vi "OAT DC Gap Estimator (1 Channel).vi"(0 "even-angle signal":cluster{"r0":dbl, "dr":dbl, "Y":dbl[]}={"r0"=0.0, "dr"=1.0, "Y"=[]} {"r0" format="%.2p"; "dr" format="%.2p"; "Y" format="%.2f"}, 1 "even-angle channel info":T2={"channel name"="", "description"="", " channel info"={"sensor sensitivity"=1000.0, "engineering units"=1, "dB reference"=1.0, "custom label"="EU", "weighting filter"=0, "pregain"=0.0}} {"channel info"."pregain" format="%.2f"; "channel info"."weighting filter" items=["Linear", "A-weighting", "B-weighting", "C-weighting", "ITU-R 468-4", "Dolby", "CCITT", "C-message", "Wb", "Wc", "Wd", "We", "Wf", "Wh", "Wj", "Wk", "Wm", "AES17 20 kHz lowpass", "AES17 40 kHz lowpass", "AES17 20 kHz highpass", "AES17 40 kHz highpass"]; "channel info"."dB reference" format="%^.1e"; "channel info"."engineering units" items=["custom..."=0, "V"=1, "A"=21, "C"=30, "pC"=31, "s"=32, "-"=29, "Pa"=2, "N"=20, "g"=3, "m/s^2"=4, "m/s"=5, "m"=6, "mm/s"=12, "mm"=13, "micron/s"=14, "micron"=15, "in/s^2"=7, "in/s"=8, "in"=9, "mil/s"=10, "mil"=11, "rad/s^2"=16, "rad/s"=17, "rad"=18, "deg/s^2"=26, "deg/s"=27, "deg"=28, "RPM"=22, "cycle/s^2"=23, "Hz"=24, "cycle"=25, "strain"=19]; "channel info"."sensor sensitivity" format="%#_5f"}, 2 "even-angle position info":T6, 3 "speed profile":T1 {"speed [RPM]" format="%.2f"; "time [s]" format="%.2f"}, 4 "gap reference [V]":dbl=inf, 5 "error in (no error)":errorcluster, 6 "x-axis selection":u16(ring)=2 items=["Time", "Revolution", "RPM"], 7 "averaging type":enum16{"Linear", "Exponential"}(ring), 8 "reset? (F)":bool, 9 "window":T7(ring), 10 "DC gap unit":u16(ring) items=["V", "EU"]) -> (14 "DC gap":T9 {"DC gap value" format="%.2f"; "time/rev/rpm" format="%.2f"}, 15 "unit labels":T8, 16 "gap position info":T6, 18 "actual gap ref [V]":dbl format="%.2f", 19 "error out":errorcluster)   [LabVIEW 2017, in "SoundVib_RefDataProcess.lvlib"]
doc: "Subtracts the gap reference from the averaged DC gap voltage of the <B>even-angle signal</B> and returns the DC gap in the selected units. The DC gap is a measurement of the movement of the shaft from the reference position to the current position. If <B>gap reference [V]</B> is unwired, the VI computes the <B>actual gap ref [V]</B> from the input signal. Wire data to the <B>even-angle signal</B> input to determine the polymorphic instance to use or manually select the instance."
uses:
  <vilib>/addons/Sound and Vibration/Order Analysis/Referece Data Processing/SoundVib_RefDataProcess.lvlib
  <vilib>/addons/Sound and Vibration/Order Analysis/Misc/OAT Position Info.ctl
  <vilib>/addons/_NISVFA/_Shared subVIs/Controls/svc_Resampled Channel Info.ctl
  <vilib>/addons/_NISVFA/_Shared subVIs/Controls/svc_Channel Info.ctl
  <vilib>/addons/_NISVFA/_Shared subVIs/Controls/svc_Engineering Units Text Ring.ctl
  <vilib>/addons/_NISVFA/_Shared subVIs/Controls/svc_Weighting Filter Text Ring.ctl
  <vilib>/addons/Sound and Vibration/Order Analysis/Tach Process/SubVIs/speed profile.ctl
  <vilib>/addons/Sound and Vibration/Order Analysis/Resample Order Tracking/SoundVib_Resampling.lvlib
  <vilib>/addons/Sound and Vibration/Order Analysis/Tach Process/SoundVib_TachProcess.lvlib
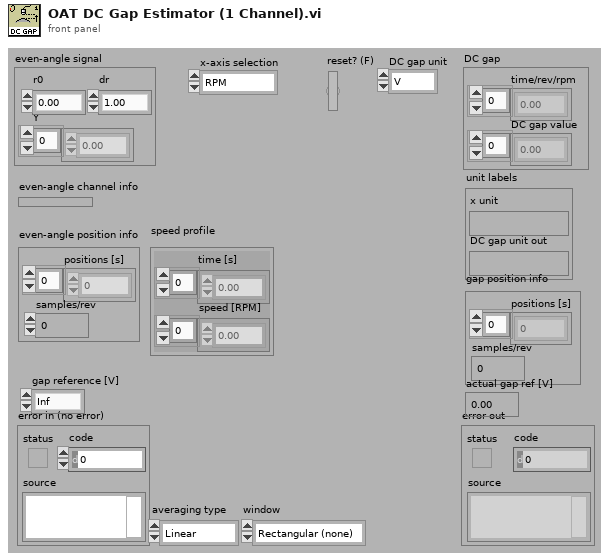
[diagram p1: front panel]
types:
  T1 = typedef "SoundVib_TachProcess.lvlib/speed profile.ctl" = cluster{"time [s]":dbl[], "speed [RPM]":dbl[]}
  T2 = typedef "svc_Resampled Channel Info.ctl" = cluster{"channel name":string, "description":string, " channel info":T3}
  T3 = typedef "svc_Channel Info.ctl" = cluster{"sensor sensitivity":dbl, "engineering units":T4, "dB reference":dbl, "custom label":string, "weighting filter":T5, "pregain":dbl}
  T4 = typedef "svc_Engineering Units Text Ring.ctl" = u16
  T5 = typedef "svc_Weighting Filter Text Ring.ctl" = u16
  T6 = typedef "OAT Position Info.ctl" = cluster{"positions [s]":dbl[], "samples/rev":dbl}
  T7 = enum16{"Rectangular (none)", "Hanning", "Low side lobe"}
  T8 = cluster{"x unit":string, "DC gap unit out":string}
  T9 = cluster{"time/rev/rpm":dbl[], "DC gap value":dbl[]}
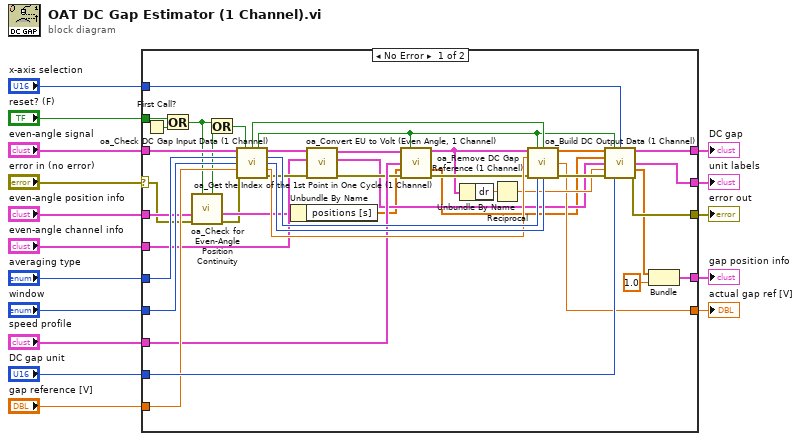
[diagram p0: block diagram]
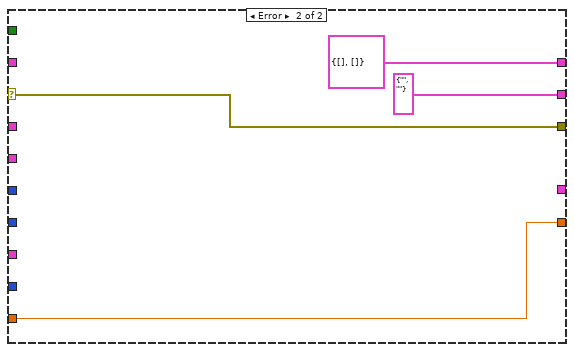
[diagram p2: hidden frame]
diagram:
  n1 = case shown="No Error" "error in (no error)" {
    selector: "error in (no error)" -> [w21 w62]
    tunnel: [w51 w62] -> w12
    tunnel: "averaging type" -> [w49 _]
    tunnel: "window" -> [w48 _]
    tunnel: "reset? (F)" -> [w58 _]
    tunnel: "gap reference [V]" -> [w45 w59]
    tunnel: "x-axis selection" -> [w54 _]
    tunnel: [w53 cluster{dbl[], dbl[]} {[], []}] -> w9
    tunnel: [w52 cluster{"X unit":string, "gap unit":string} {"X unit"="", "gap unit"=""} ("unit labels")] -> w8
    tunnel: "DC gap unit" -> [w50 _]
    tunnel: [w39 w59] -> w6
    tunnel: [w36 _] -> w5
    tunnel: "even-angle signal" -> [w35 _]
    tunnel: "even-angle channel info" -> [w24 _]
    tunnel: "speed profile" -> [w34 _]
    tunnel: "even-angle position info" -> [w23 _]
    frame No Error {
      n2 = First Call?() -> (First Call?: T/F=w57:bool)
      n3 = Or(x=w58, y=w57) -> (x .or. y?=w18:bool)
      n4 = call <vilib>:"oa_Check for Even-Angle Position Continuity.vi"("reset in"=w18, "error in (no error)"=w21, "even-angle position info"=w23) -> ("error out"=w20:errorcluster, "even-angle position info dup"=w22:T6, "position not continuous"=w19:bool)  [unwired: 6 in]
      n5 = Or(x=w18, y=w19) -> (x .or. y?=w17:bool)
      n6 = call <vilib>:"oa_Check DC Gap Input Data (1 Channel).vi"("even angle signal"=w35, "reset"=w17, "averaging type"=w49, "window"=w48, "DC gap reference [V]"=w45, "error in (no error)"=w20) -> ("DC ref changed?"=w28:bool, "reset?"=w27:bool, "even angle signal"=w33:cluster{"r0":dbl, "dr":dbl, "Y":dbl[]}, "averaging type out"=w47:enum16{"Linear", "Exponential"}, "window out"=w46:T7, "DC gap reference [V] out"=w44:dbl, "error out"=w32:errorcluster)  [unwired: 3 in]
      n7 = Unbundle By Name(w22) -> ("positions [s]"=w26:dbl[])
      n8 = call <vilib>:"oa_Convert EU to Volt (Even Angle, 1 Channel).vi"("error in (no error)"=w32, "even angle channel info"=w24, "even angle signal"=w33) -> ("error out"=w31:errorcluster, "channel info"=w29:T3, "even angle signal"=w30:cluster{"r0":dbl, "dr":dbl, "Y":dbl[]})  [unwired: 6 in]
      n9 = call <vilib>:"oa_Get the Index of the 1st Point in One Cycle (1 Channel).vi"("resampled signal"=w30, "reset? (True)"=w27, "speed profile"=w34, "interpolated pulse positions"=w26, "error in (no error)"=w31) -> ("resampled signal out"=w42:cluster{"r0":dbl, "dr":dbl, "Y":dbl[]}, "interpolated pulse positions out"=w25:dbl[], "error out"=w43:errorcluster)  [unwired: 8 in]
      n10 = Unbundle By Name(w42) -> ("dr"=w41:dbl)
      n11 = Reciprocal(x=w41) -> (1/x=w40:dbl)
      n12 = call <vilib>:"oa_Remove DC Gap Reference (1 Channel).vi"("resampled signal"=w42, "reset?"=w27, "DC ref changed?"=w28, "DC gap reference [V]"=w44, "error in"=w43, "averaging type"=w47, "window"=w46) -> ("DC value out"=w56:dbl[], "actual gap ref"=w39:dbl, "error out"=w55:errorcluster)  [unwired: 6 in]
      n13 = call <vilib>:"oa_Build DC Output Data (1 Channel).vi"("DC value out"=w56, "reset? (True)"=w27, "X axis selection"=w54, "start points"=w25, "channel info"=w29, "samples/rev"=w40, "error in (no error)"=w55, "DC gap unit"=w50) -> ("DC Gap"=w53:cluster{"X":dbl[], "Y":dbl[]}, "unit labels"=w52:cluster{"X unit":string, "gap unit":string}, "DC gap positions [s]"=w38:dbl[], "error out"=w51:errorcluster)  [unwired: 4 in]
      n14 = Bundle("DC gap positions [s]"=w38, 1.0) -> (w36:cluster{"DC gap positions [s]":dbl[], dbl})  [unwired: 1 in]
    }
    frame Error {
    }
  }
  "error out" <- w12
  "DC gap" <- w9
  "unit labels" <- w8
  "gap position info" <- w5
  "actual gap ref [V]" <- w6
